vi "Begin ServerStreamTemplate.vi"(8 "error in":errorcluster, 10 "Request Data":cluster{"Numeric":dbl}, 11 "gRPC ID":T1) -> (0 "error out":errorcluster, 2 "Call Id Out":T1, 3 "gRPC ID out":T1)   [LabVIEW 2019, in "Client Template.lvlib"]
uses:
  <vilib>/gRPC/LabVIEW gRPC Library/Server API/typeDefs/grpcId.ctl
  Client Template.lvlib
  59bd46bd-855a-43b3-a0b3-6a244c6a481b.vi
  <vilib>/gRPC/LabVIEW gRPC Library/gprc-lvsupport-release.lvlib
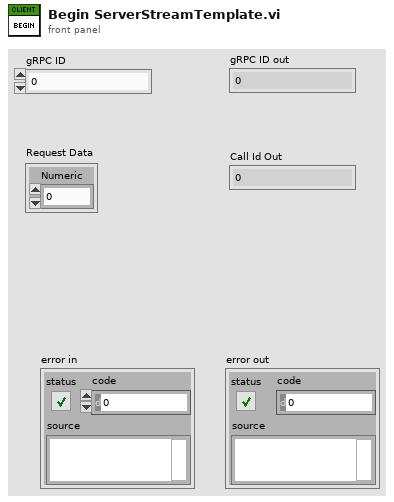
[diagram p1: front panel]
types:
  T1 = typedef "gprc-lvsupport-release.lvlib/grpcId.ctl" = u64
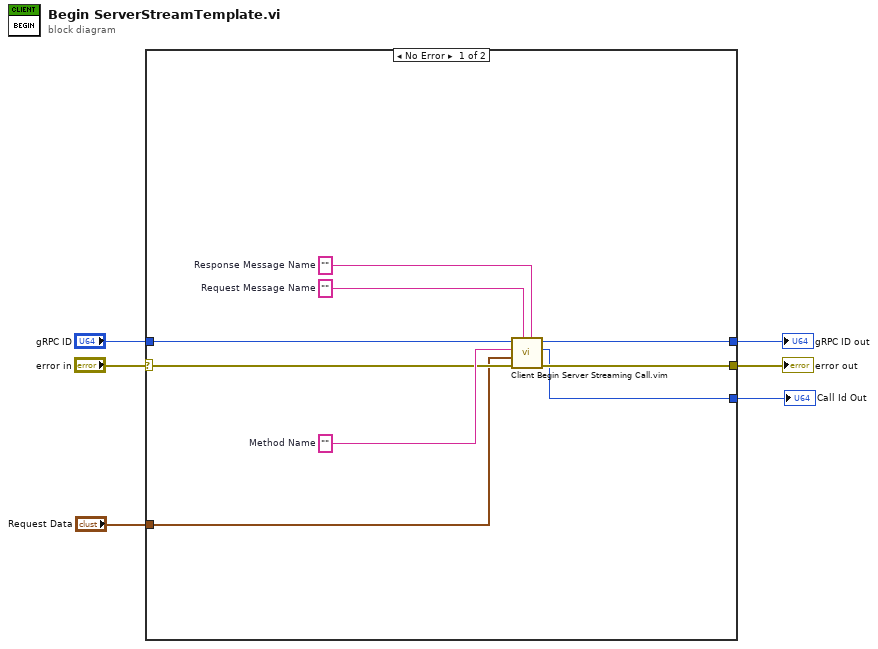
[diagram p0: block diagram]
diagram:
  n1 = case shown="No Error" "error in" {
    selector: "error in" -> [w12 w16]
    tunnel: [w11 w16] -> w5
    tunnel: "gRPC ID" -> [w10 w17]
    tunnel: [w9 w17] -> w3
    tunnel: [w8 _] -> w2
    tunnel: "Request Data" -> [w7 _]
    frame No Error {
      w13 = ""  # Response Message Name
      w14 = ""  # Request Message Name
      w15 = ""  # Method Name
      n2 = call "Client Begin Server Streaming Call.vim"("Response Message Name"=w13, "Request Message Name"=w14, "error in (no error)"=w12, "Request Data"=w7, "Method Name"=w15, "Client Ref"=w10) -> ("error out"=w11:errorcluster, "Call Id Out"=w8:u64, "Client Ref Out"=w9:u64)  [unwired: 3 in]
    }
    frame Error {
    }
  }
  "error out" <- w5
  "gRPC ID out" <- w3
  "Call Id Out" <- w2
